vi "PA -Move to absolute position.vi"(4 "Move to absolute\nposition - set":dbl, 6 "error in":errorcluster, 7 "Action":bool, 8 "Axis #":i8=1 min=1 max=6 step=1, 9 "Address / Port":i16=1 min=1 max=31 step=1) -> (0 "error out":errorcluster, 1 "Query current actual\nposition - read":string, 2 "Axis # dup":i8=1 min=1 max=6 step=1, 3 "Address / Port dup":i16=1 min=1 max=31 step=1)   [LabVIEW 2014]
panel:
  # "Read"
  # "Write"
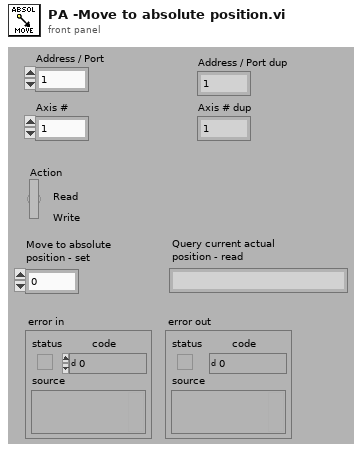
[diagram p1: front panel]
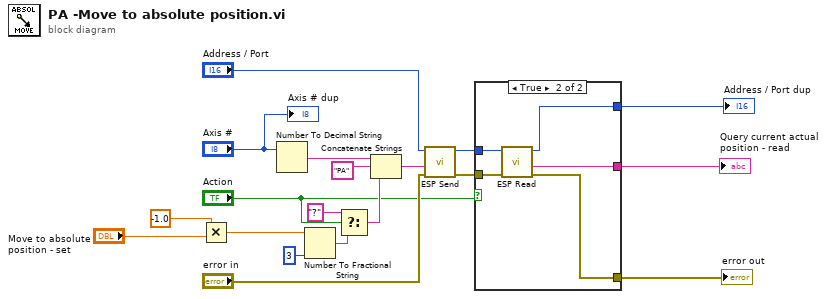
[diagram p0: block diagram]
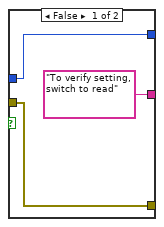
[diagram p2: hidden frame]
diagram:
  n1 = Multiply(x=-1.0, y="Move to absolute\nposition - set") -> (x*y=w1:dbl)
  n2 = Number To Decimal String(number="Axis #") -> (decimal integer string=w18:string)  [unwired: 1 in]
  n3 = Number To Fractional String(number=w1, precision (6)=i16 3) -> (F-format string=w14:string)  [unwired: 2 in]
  n4 = Select(t="?", s="Action", f=w14) -> (s? t:f=w15:string)
  n5 = Concatenate Strings(w18, "PA" ("Substring"), w15) -> (w16:string)
  n6 = call "ESP Send.vi"("error in"="error in", "Command String"=w16, "Address / Port"="Address / Port") -> ("error out"=w9:errorcluster, "Address / Port dup"=w6:i16)  [unwired: 3 in]
  n7 = case shown="True" "Action" {
    tunnel: w6 -> [w20 w27]
    tunnel: w9 -> [w22 w26]
    tunnel: [w22 w25] -> w8
    tunnel: ["To verify setting, switch to read" w24] -> w7
    tunnel: [w20 w23] -> w5
    frame False {
    }
    frame True {
      n8 = call "ESP Read.vi"("error in"=w26, "Address / Port"=w27) -> ("error out"=w25:errorcluster, "Response String"=w24:string, "Address / Port dup"=w23:i16)  [unwired: 3 in]
    }
  }
  "error out" <- w8
  "Query current actual\nposition - read" <- w7
  "Address / Port dup" <- w5
  "Axis # dup" <- "Axis #"
